vi "Teardown.vi"(11 "jettl Msg Teardown in":refnum<class "jettl Msg Teardown.lvclass">) -> (3 "jettl Msg Teardown out":refnum<class "jettl Msg Teardown.lvclass">)   [LabVIEW 2021, in "jettl Msg Teardown.lvlib" / "jettl Msg Teardown.lvclass"]
uses:
  jettl Msg Teardown.lvclass
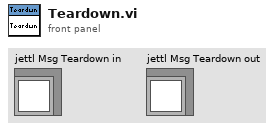
[diagram p1: front panel]
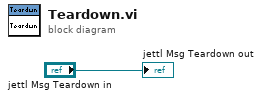
[diagram p0: block diagram]
diagram:
  "jettl Msg Teardown out" <- "jettl Msg Teardown in"
